vi "RecieveFrame.vi"(8 "error in":errorcluster, 11 "FrameOut session in":refnum<k21>) -> (0 "error out":errorcluster, 1 "LIN communication state":T1 {"communication state" items=["Idle", "Active", "Inactive"]; "fault code" format="%08x"; "last error" items=["None", "Unknown ID", "Form", "Framing", "Readback", "Timeout", "Checksum"]}, 2 "DataBytes":string[](array[string]), 3 "session out":refnum<k21>)   [LabVIEW 2018]
uses:
  <vilib>/xnet/xnet.llb/XNET LIN Comm.ctl
  <vilib>/xnet/xnet.llb/XNET LIN Comm State.ctl
  <vilib>/xnet/xnet.llb/XNET LIN Last Err.ctl
  <vilib>/xnet/xnet.llb/XNET Read (State LIN Comm).vi
  <vilib>/xnet/xnet.llb/XNET Read (Frame LIN).vi
  <vilib>/regexp/Match Regular Expression.xnode
panel:
  out "element":string[](array[string])
  out "Finish":bool
  out "MulFrame?":bool
  out "GetKey?":bool
  out "Error?":bool
  out "匹配后偏移量":i32
  out "DataBytes 2":u8[](array[numeric]) format="%.0x"
  in  "Frame 2":string
  out "Frame":string[][](array[string])
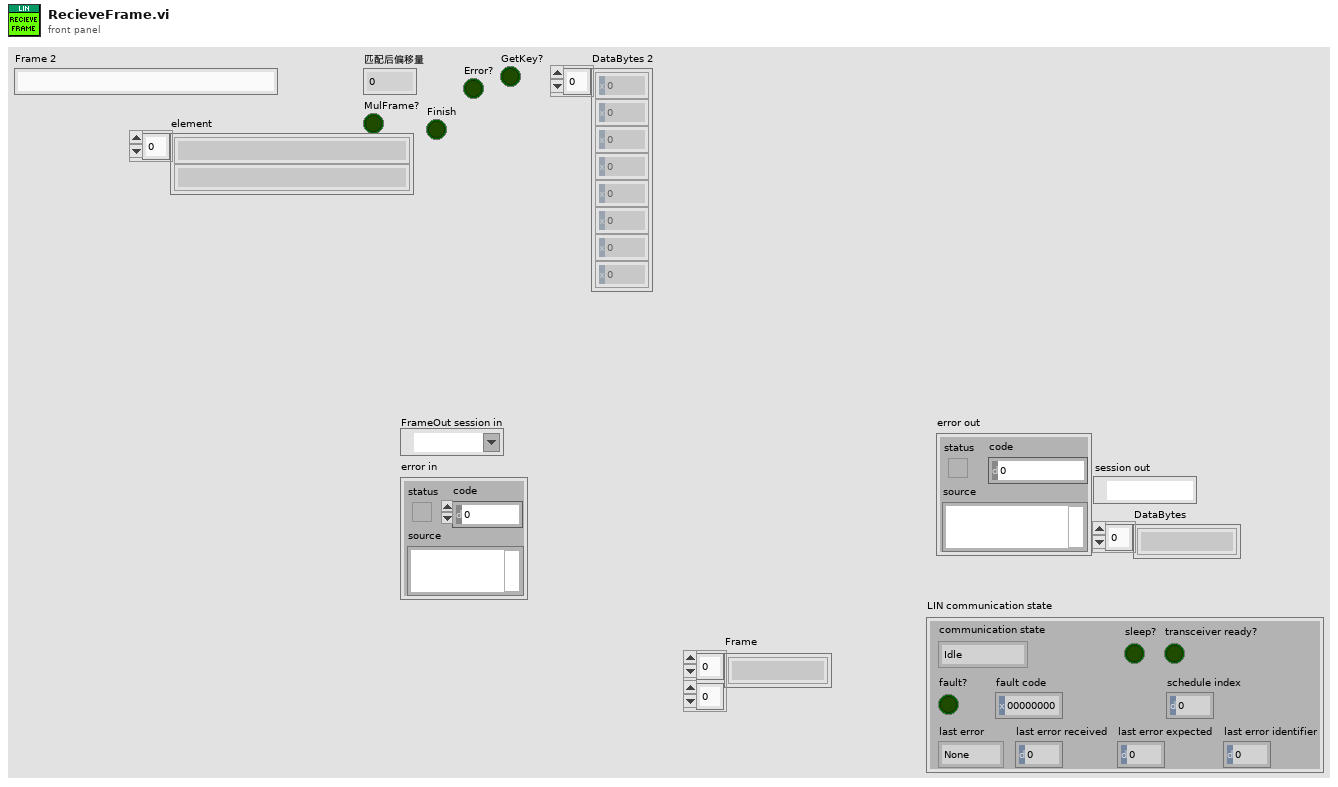
[diagram p1: front panel]
types:
  T1 = typedef "XNET LIN Comm.ctl" = cluster{"fault code":i32, "fault?":bool, "communication state":T2, "last error":T3, "last error received":u8, "last error expected":u8, "last error identifier":u8, "sleep?":bool, "transceiver ready?":bool, "schedule index":u8}
  T2 = typedef "XNET LIN Comm State.ctl" = u8
  T3 = typedef "XNET LIN Last Err.ctl" = u8
  T4 = typedef "XNET Frame LIN.ctl" = cluster{"timestamp":timestamp, "payload":u8[], "identifier":u32, "type":T5, "event ID":u8, "event slot?":bool, "echo?":bool}
  T5 = typedef "XNET Frame Type LIN.ctl" = u8
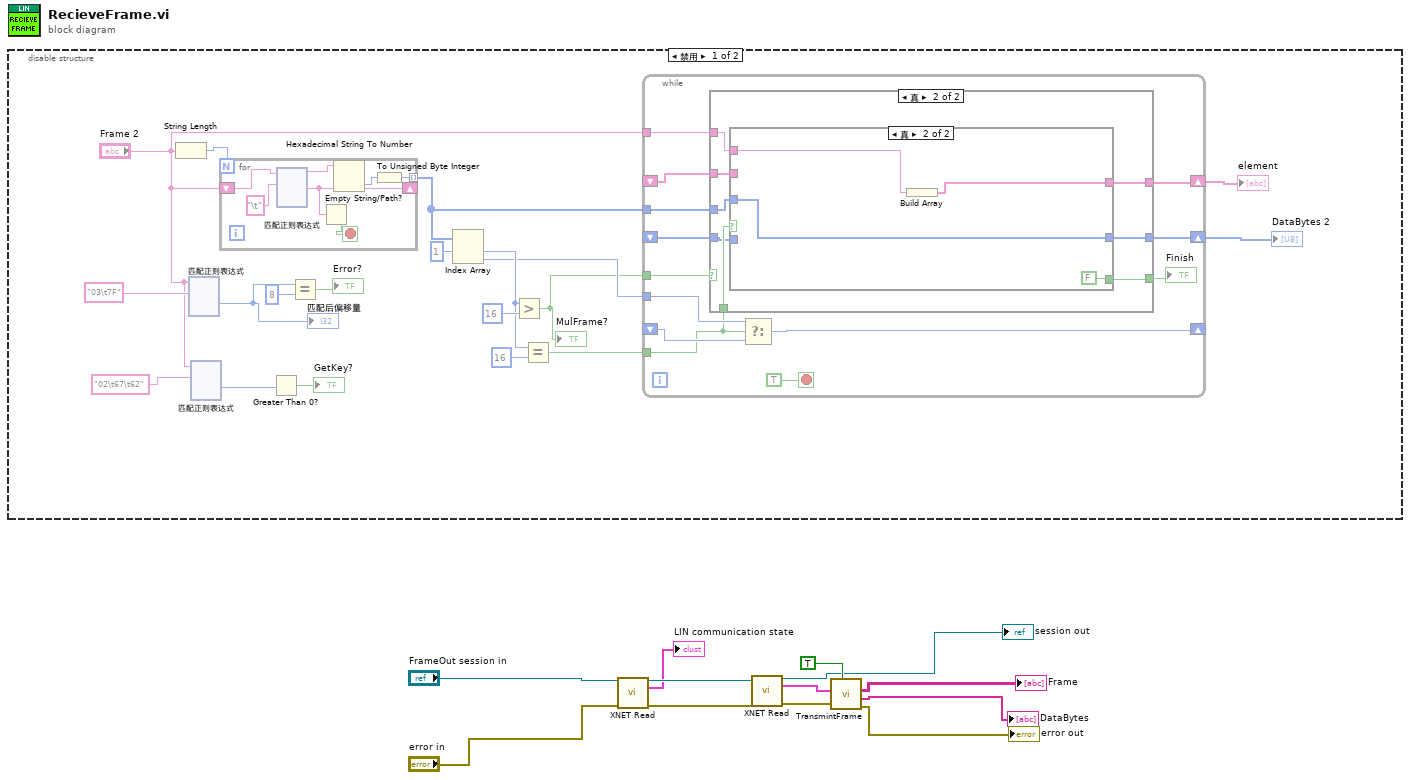
[diagram p0: block diagram]
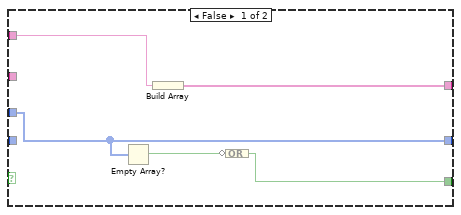
[diagram p2: hidden frame]
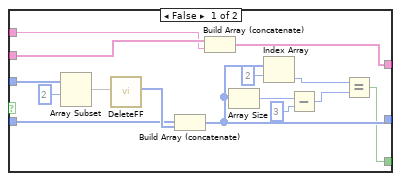
[diagram p3: hidden frame]
diagram:
  n1 = disable-structure shown="禁用" {
    frame Disabled {
      n2 = String Length(string="Frame 2") -> (length=w31:i32)
      n3 = xnode "匹配正则表达式"("input string"="Frame 2", "regular expression"="03\t7F" ("Frame")) -> ("offset past match"=w29:i32)  [unwired: 4 in, 4 out]
      "匹配后偏移量" <- w29
      n4 = xnode "匹配正则表达式"("input string"="Frame 2", "regular expression"="02\t67\t62" ("正则表达式")) -> ("offset past match"=w24:i32)  [unwired: 4 in, 4 out]
      n5 = for {
        N: w31 -> [_]
        shift-right: [w309] -> _
        shift-left: "Frame 2" -> [w311]
        tunnel: [w305] -> w16 mode=indexing
        stop <- w308 stop-if-true
        n6 = xnode "匹配正则表达式"("input string"=w311, "regular expression"="\t" ("正则表达式")) -> ("before match"=w306:string, "after match"=w309:string)  [unwired: 4 in, 3 out]
        n7 = Empty String/Path?(string/path=w309) -> (empty?=w308:bool)
        n8 = Hexadecimal String To Number(string=w306) -> (number=w307:u32)  [unwired: 2 in, 1 out]
        n9 = To Unsigned Byte Integer(number=w307) -> (unsigned 8bit integer=w305:u8)
      }
      n10 = Greater Than 0?(x=w24) -> (x > 0?=→"GetKey?":bool)
      n11 = Equal?(x=w29, y=8) -> (x = y?=→"Error?":bool)
      n12 = Index Array(array=w16, index #1=1 ("索引")) -> (element #1=w21:u8, element #2=w18:u8)  [unwired: 1 in]
      n13 = Greater?(x=w21, y=u8 16) -> (0:w17:bool)
      "MulFrame?" <- w17
      n14 = Equal?(x=w21, y=u8 16) -> (x = y?=w19:bool)
      n15 = while {
        tunnel: w19 -> [w39]
        shift-right: [w43] -> _
        shift-left: _ -> [w41]
        tunnel: w18 -> [w42]
        tunnel: w17 -> [w40]
        tunnel: w16 -> [w38]
        shift-right: [w37] -> w15
        shift-left: _ -> [w36]
        tunnel: "Frame 2" -> [w34]
        shift-right: [w33] -> w13
        shift-left: _ -> [w32]
        stop <- TRUE stop-if-true
        n16 = case shown="真" w40 {
          tunnel: w39 -> [_ w57]
          tunnel: w38 -> [w49 w55]
          tunnel: [w49 w56] -> w37
          tunnel: w36 -> [_ w54]
          tunnel: [w47 w53] -> w35
          tunnel: w34 -> [w46 w52]
          tunnel: [w45 w51] -> w33
          tunnel: w32 -> [_ w50]
          frame False {
            n17 = Empty Array?(array=w49) -> (empty?=w48:bool)
            n18 = Build Array(w46) -> (w45:string[])
            n19 = Compound Arithmetic op=OR ("复合运算")(invert w48) -> (w47:bool)
          }
          frame True {
            n20 = case shown="真" w57 {
              tunnel: [w65 w76] -> w56
              tunnel: w55 -> [w72 w76]
              tunnel: w54 -> [w68 _]
              tunnel: [w61 FALSE] -> w53
              tunnel: w52 -> [w59 w74]
              tunnel: [w58 w73] -> w51
              tunnel: w50 -> [w60 _]
              frame False {
                n21 = Array Subset(array=w72, index=2 ("索引")) -> (w70:u8[])  [unwired: 1 in]
                n22 = call "DeleteFF.vi"("Data"=w70) -> ("Data out"=w69:u8[])  [unwired: 10 in]
                n23 = Build Array (concatenate)(w68, w69) -> (w65:u8[])
                n24 = Build Array (concatenate)(w60, w59) -> (w58:string[])
                n25 = Array Size(array=w65) -> (size(s)=w67:i32)
                n26 = Index Array(array=w65, index=2 ("索引")) -> (element=w63:u8)
                n27 = Subtract(x=w67, y=3) -> (x-y=w62:i32)
                n28 = Equal?(x=w63, y=w62) -> (x = y?=w61:bool)
              }
              frame True {
                n29 = Build Array(w74) -> (w73:string[])
              }
            }
          }
        }
        "Finish" <- w35
        n30 = Select(t=w42, s=w39, f=w41) -> (s? t:f=w43:u8)
      }
      "DataBytes 2" <- w15
      "element" <- w13
    }
    frame Enabled {
    }
  }
  n31 = call-poly <vilib>:"XNET Read.vi"("session in"="FrameOut session in", "error in (no error)"="error in") -> ("session out"=w9:refnum<k21>, "LIN comm"=→"LIN communication state":T1, "error out"=w10:errorcluster)  [unwired: 11 out]
  n32 = call-poly <vilib>:"XNET Read.vi"("session in"=w9, "error in (no error)"=w10) -> ("session out"=→"session out":refnum<k21>, "data"=w6:T4[], "error out"=w5:errorcluster)  [unwired: 11 out]
  n33 = call "TransmintFrame.vi"("Hex and Dec"=TRUE ("Hexadecimal?"), "error in (no error)"=w5, "data"=w6) -> ("error out"=→"error out":errorcluster, "DataByte"=→"DataBytes":string[], "Output Array"=→"Frame":string[][])  [unwired: 6 in]
